vi "get head status.vi"(8 "error in (no error)":errorcluster, 11 "head":u16) -> (0 "error out":errorcluster, 3 "function return":u16)   [LabVIEW 2015, in "SCANalone4x64.lvlib"]
doc: "__declspec(dllimport) unsigned short __stdcall get_head_status(unsigned short head);"
uses:
  <userlib>/SCANalone4x64/SCANalone4x64.lvlib
  <userlib>/SCANalone4x64/SCANalone4x64.dll
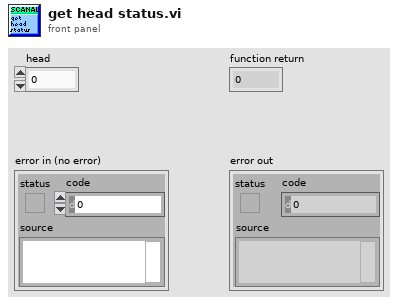
[diagram p1: front panel]
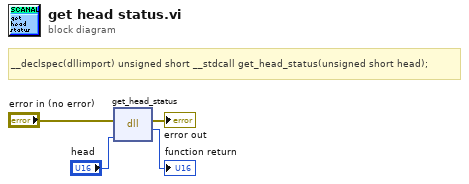
[diagram p0: block diagram]
diagram:
  # "__declspec(dllimport) unsigned short __stdcall get_head_status(unsigned short head);"
  n1 = dll-call lib="C:/Program Files/National Instruments/LabVIEW 2015/user.lib/SCANalone4x64/SCANalone4x64.*" fn="get_head_status"(error in="error in (no error)", "head"="head") -> (error out=→"error out":errorcluster, →"function return":u16)  [unwired: 3 in, 1 out]
